vi "Trafic_Lights.vi"() -> ()   [LabVIEW 2019]
uses:
  Traffic_Lights_states.ctl
panel:
  out "String":string="Stelios"
  out "Red":bool
  out "Yellow":bool
  out "Green":bool
  in  "stop":bool
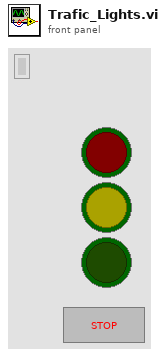
[diagram p1: front panel]
types:
  T1 = typedef "Traffic_Lights_states.ctl" = enum16{"Green", "Yellow", "Red"}
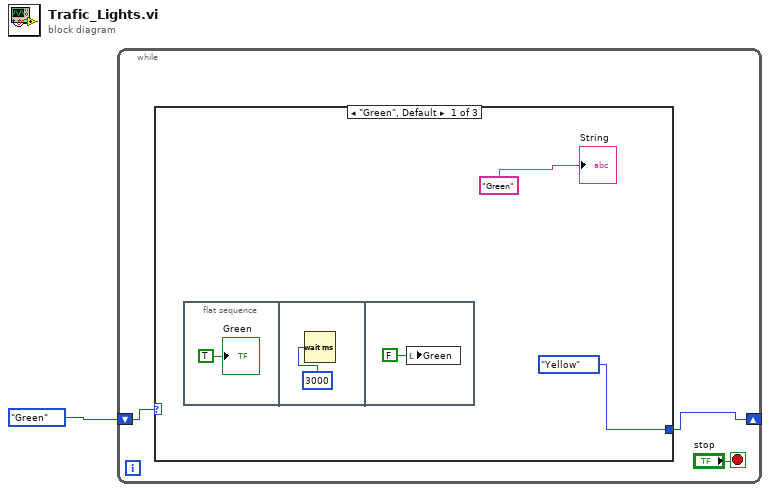
[diagram p0: block diagram]
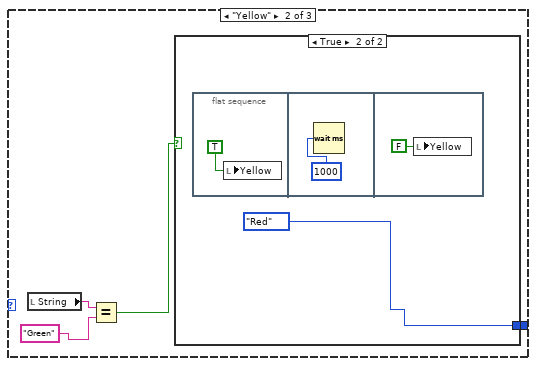
[diagram p2: hidden frame]
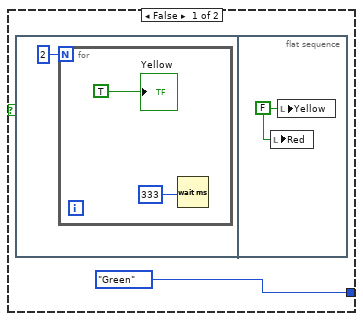
[diagram p3: hidden frame]
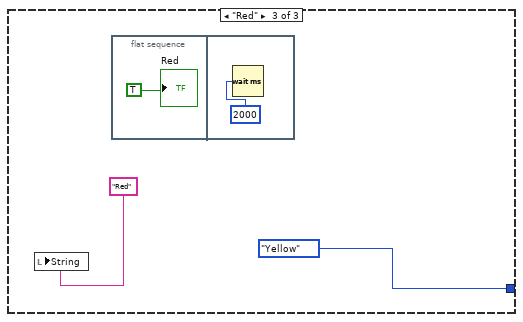
[diagram p4: hidden frame]
diagram:
  n1 = while {
    shift-right: [w3] -> _
    shift-left: Traffic_Lights_states."Green" -> [w2]
    stop <- "stop" stop-if-true
    n2 = case shown="\"Green\", Default" w2 {
      tunnel: [Traffic_Lights_states."Yellow" w11 Traffic_Lights_states."Yellow"] -> w3
      frame "Green", Default {
        n3 = flat-sequence {
          frame #0 {
            "Green" <- TRUE ("Green")
          }
          frame #1 {
            n4 = Wait (ms)(milliseconds to wait=u32 3000 ("millisecond timer value")) -> ()  [unwired: 1 out]
          }
          frame #2 {
            n5 = local write "Green"(FALSE ("Green")) -> ()
          }
        }
        "String" <- "Green"
      }
      frame "Yellow" {
        n6 = local read "String"() -> (w12:string)
        n7 = Equal?(x=w12, y="Green") -> (x = y?=w10:bool)
        n8 = case shown="True" w10 {
          tunnel: [Traffic_Lights_states."Green" Traffic_Lights_states."Red"] -> w11
          frame False {
            n9 = flat-sequence {
              frame #0 {
                n10 = for {
                  N: 2 -> [_]
                  n11 = Wait (ms)(milliseconds to wait=u32 333 ("millisecond timer value")) -> ()  [unwired: 1 out]
                  "Yellow" <- TRUE ("Green")
                }
              }
              frame #1 {
                w18 = FALSE ("Green")
                n12 = local write "Red"(w18) -> ()
                n13 = local write "Yellow"(w18) -> ()
              }
            }
          }
          frame True {
            n14 = flat-sequence {
              frame #0 {
                n15 = local write "Yellow"(TRUE ("Green")) -> ()
              }
              frame #1 {
                n16 = Wait (ms)(milliseconds to wait=u32 1000 ("millisecond timer value")) -> ()  [unwired: 1 out]
              }
              frame #2 {
                n17 = local write "Yellow"(FALSE ("Green")) -> ()
              }
            }
          }
        }
      }
      frame "Red" {
        n18 = local write "String"("Red") -> ()
        n19 = flat-sequence {
          frame #0 {
            "Red" <- TRUE ("Green")
          }
          frame #1 {
            n20 = Wait (ms)(milliseconds to wait=u32 2000 ("millisecond timer value")) -> ()  [unwired: 1 out]
          }
        }
      }
    }
  }
